vi "Newport PM Stand Alone Test.vi"() -> ()   [LabVIEW 2017]
uses:
  Device State Control.ctl
panel:
  out "Sample Count":i32
  out "Error":bool
  out "Readings Being Updated":bool
  out "2936R error out":errorcluster
  in  "USB Address":i32=1
  in  "Time Interval":dbl=0.5 caption="Delay Time (s)" format="%_3g"
  in  "stop":bool
  out "Ch2, W":dbl format="%_6e"
  out "CH1, W":dbl format="%_6e"
  in  "PowerMeter 2936R Settings":T1={"Wavelength nm"=600, "Range Select"=0, "Mode"=0, "Unit Select"=2, "Auto Select"=1, "Analog Filter"=0, "Digital Filter (int. 0 to 10000)"=0, "Filter"=0} {"Filter" items=["No filtering", "Analog filter", "Digital filter", "Analog and Digital filter"]; "Digital Filter (int. 0 to 10000)" min=0 max=10000; "Analog Filter" items=["None", "250 kHz", "12.5 kHz", "1 kHz", "5 kHz"]; "Auto Select" items=["Manual Range", "Auto Range"]; "Unit Select" items=["Amps", "Volts", "Watts", "Watts/cm2", "Joules", "Joules/cm2", "dBm"]; "Mode" items=["CW Cont.", "DC Single", "Integrate", "Peak-to-Peak Cont.", "Peak-to-Peak Single", "Pulse Continuous", "Pulse Single", "RMS"]; "Range Select" items=["Range 0", "Range 1", "Range 2", "Range 3", "Range 4", "Range 5", "Range 6", "Range 7"]; "Wavelength nm" min=0}
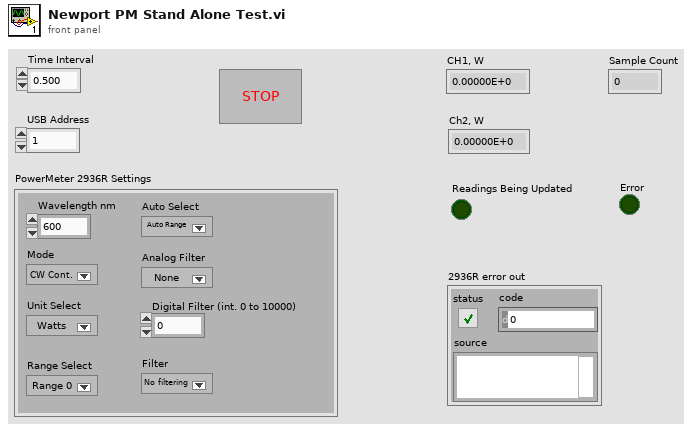
[diagram p1: front panel]
types:
  T1 = cluster{"Wavelength nm":i32, "Range Select":i32, "Mode":i32, "Unit Select":i32, "Auto Select":i32, "Analog Filter":i32, "Digital Filter (int. 0 to 10000)":i32, "Filter":i32}
  T2 = typedef "Device State Control.ctl" = enum16{"Open", "Close", "Clear", "Set", "Reset", "Read", "Write", "Call"}
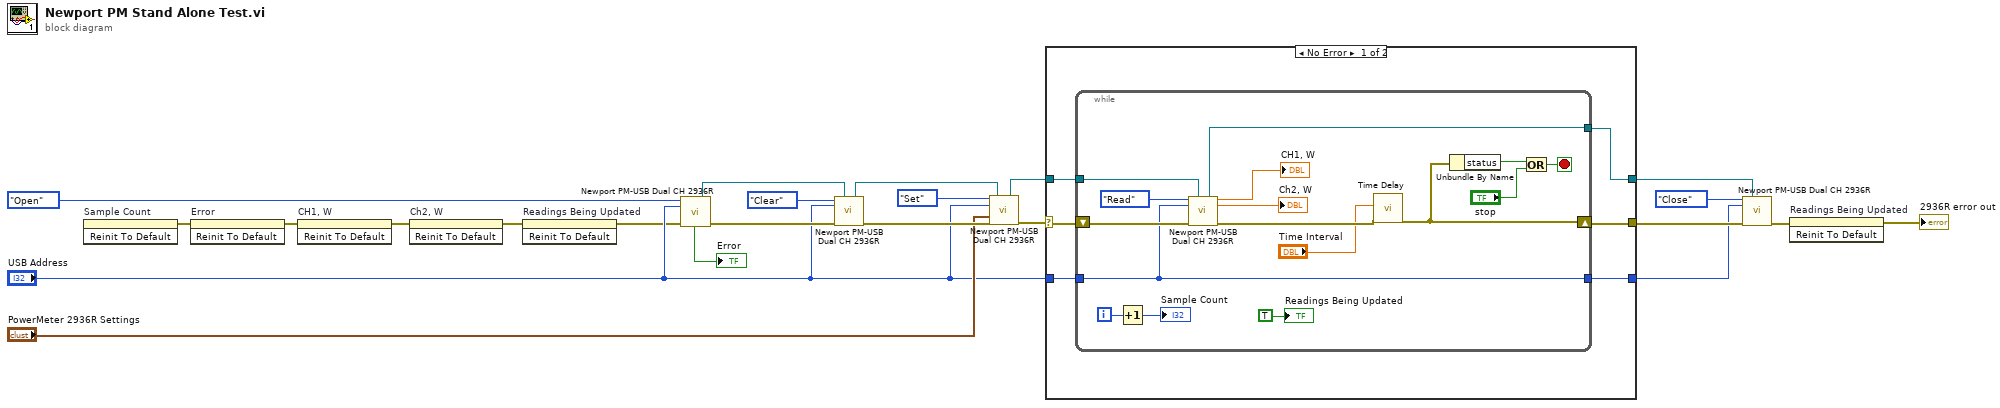
[diagram p0: block diagram]
diagram:
  n1 = invoke on="Sample Count" class="DigNum (strict)" method="Reinit To Default"() -> (error out=w1:errorcluster)  [unwired: 3 in, 2 out]
  n2 = invoke on="Error" class="Bool (strict)" method="Reinit To Default"(error in=w1) -> (error out=w2:errorcluster)  [unwired: 2 in, 2 out]
  n3 = invoke on="CH1, W" class="DigNum (strict)" method="Reinit To Default"(error in=w2) -> (error out=w4:errorcluster)  [unwired: 2 in, 2 out]
  n4 = invoke on="Ch2, W" class="DigNum (strict)" method="Reinit To Default"(error in=w4) -> (error out=w5:errorcluster)  [unwired: 2 in, 2 out]
  n5 = invoke on="Readings Being Updated" class="Bool (strict)" method="Reinit To Default"(error in=w5) -> (error out=w8:errorcluster)  [unwired: 2 in, 2 out]
  n6 = call "Newport PM-USB Dual CH 2936R.vi"("Device State Control"=Device_State_Control."Open", "USB Address"="USB Address", "2936R error in"=w8) -> ("2936R Ref Out"=w22:refnum<k24>, "Error"=→"Error":bool, "2936R error out"=w17:errorcluster)  [unwired: 5 in, 5 out]
  n7 = call "Newport PM-USB Dual CH 2936R.vi"("Device State Control"=Device_State_Control."Clear", "2936R Ref In"=w22, "USB Address"="USB Address", "2936R error in"=w17) -> ("2936R Ref Out"=w20:refnum<k24>, "2936R error out"=w16:errorcluster)  [unwired: 4 in, 6 out]
  n8 = call "Newport PM-USB Dual CH 2936R.vi"("Device State Control"=Device_State_Control."Set", "2936R Ref In"=w20, "USB Address"="USB Address", "PowerMeter 2936R Settings"="PowerMeter 2936R Settings", "2936R error in"=w16) -> ("2936R Ref Out"=w18:refnum<k24>, "2936R error out"=w9:errorcluster)  [unwired: 3 in, 6 out]
  n9 = case shown="No Error" w9 {
    selector: w9 -> [w24 w47]
    tunnel: w18 -> [w29 w48]
    tunnel: [w28 w47] -> w14
    tunnel: "USB Address" -> [w27 w46]
    tunnel: [w26 w46] -> w12
    tunnel: [w25 w48] -> w10
    frame No Error {
      n10 = while {
        tunnel: w29 -> [w45]
        tunnel: w27 -> [w34]
        shift-right: [w38] -> w28
        shift-left: w24 -> [w40]
        tunnel: [w34] -> w26
        tunnel: [w33] -> w25
        i -> [w31]
        stop <- w35 stop-if-true
        n11 = Increment(x=w31) -> (x+1=→"Sample Count":i32)
        n12 = call "Newport PM-USB Dual CH 2936R.vi"("Device State Control"=Device_State_Control."Read", "2936R Ref In"=w45, "USB Address"=w34, "2936R error in"=w40) -> ("2936R Ref Out"=w33:refnum<k24>, "CH1, W"=→"CH1, W":dbl, "Ch2, W"=→"Ch2, W":dbl, "2936R error out"=w41:errorcluster)  [unwired: 4 in, 4 out]
        n13 = call "Time Delay"("error in (no error)"=w41, "Delay Time (s)"="Time Interval") -> ("error out"=w38:errorcluster)  [unwired: 9 in]
        n14 = Unbundle By Name(w38) -> ("status"=w37:bool)
        n15 = Or(x=w37, y="stop") -> (x .or. y?=w35:bool)
        "Readings Being Updated" <- TRUE ("Readings Being Updated")
      }
    }
    frame Error {
    }
  }
  n16 = call "Newport PM-USB Dual CH 2936R.vi"("Device State Control"=Device_State_Control."Close", "2936R Ref In"=w10, "USB Address"=w12, "2936R error in"=w14) -> ("2936R error out"=w7:errorcluster)  [unwired: 4 in, 7 out]
  n17 = invoke on="Readings Being Updated" class="Bool (strict)" method="Reinit To Default"(error in=w7) -> (error out=→"2936R error out":errorcluster)  [unwired: 2 in, 2 out]
